vi "graphrangev2.vi"(1 "input tone start power (dBm)":dbl[](array[numeric]), 2 "input tone end power (dBm)":dbl[](array[numeric])) -> (0 "Bottom":dbl, 3 "Top":dbl)   [LabVIEW 2009]
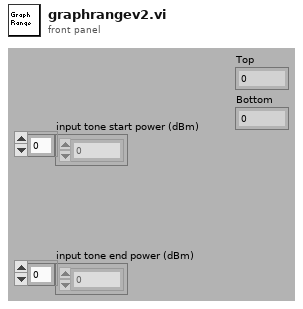
[diagram p1: front panel]
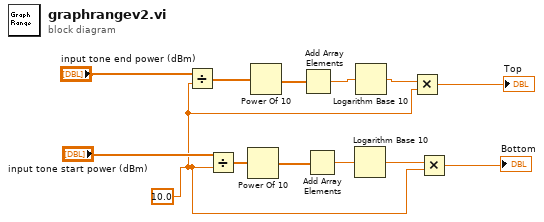
[diagram p0: block diagram]
diagram:
  w5 = 10.0
  n1 = Divide(x="input tone end power (dBm)", y=w5) -> (x/y=w13:dbl[])
  n2 = Divide(x="input tone start power (dBm)", y=w5) -> (x/y=w12:dbl[])
  n3 = Power Of 10(x=w12) -> (10^x=w9:dbl[])
  n4 = Power Of 10(x=w13) -> (10^x=w10:dbl[])
  n5 = Add Array Elements(numeric array=w10) -> (sum=w2:dbl)
  n6 = Add Array Elements(numeric array=w9) -> (sum=w7:dbl)
  n7 = Logarithm Base 10(1:w7) -> (0:w6:dbl)
  n8 = Logarithm Base 10(1:w2) -> (0:w1:dbl)
  n9 = Multiply(x=w1, y=w5) -> (x*y=→"Top":dbl)
  n10 = Multiply(x=w6, y=w5) -> (x*y=→"Bottom":dbl)
